vi "Excel_Insert_Text.vi"(0 "worksheet":refnum<k7>, 1 "font":T1 {"font size" format="%0.2f"; "strike through" items=["Unchanged", "Yes", "No"]; "underline" items=["Unchanged", "Yes", "No"]; "italic" items=["Unchanged", "Yes", "No"]; "bold" items=["Unchanged", "Yes", "No"]}, 3 "from template?":bool, 7 "value":string, 11 "error in (no error)":errorcluster, 12 "row":i32, 13 "column":i32, 14 "name":string) -> (15 "error out":errorcluster)   [LabVIEW 2017, in "NI_ReportGenerationToolkit.lvlib"]
uses:
  <vilib>/addons/_office/NI_ReportGenerationToolkit.lvlib
  <vilib>/addons/_office/_exclsub.llb/font.ctl
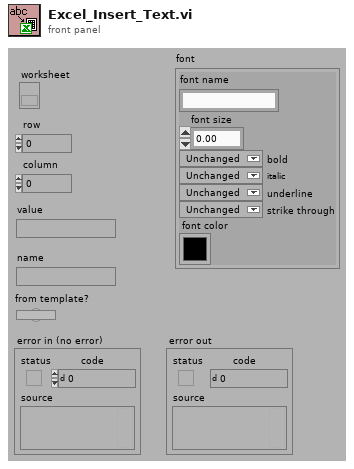
[diagram p1: front panel]
types:
  T1 = typedef "NI_ReportGenerationToolkit.lvlib/font.ctl" = cluster{"font name":string, "font size":dbl, "bold":u16, "italic":u16, "underline":u16, "strike through":u16, "font color":u32}
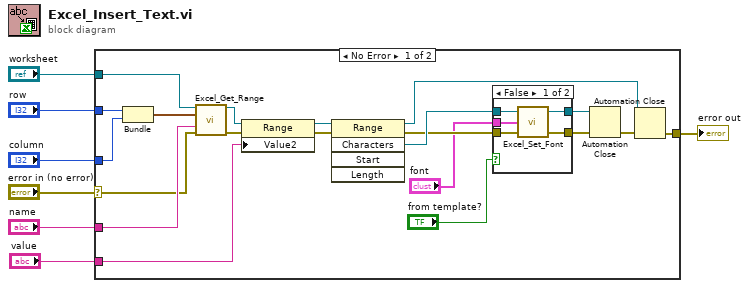
[diagram p0: block diagram]
diagram:
  n1 = case shown="No Error" "error in (no error)" {
    selector: "error in (no error)" -> [w9 w35]
    tunnel: "value" -> [w27 _]
    tunnel: [w26 w35] -> w6
    tunnel: "worksheet" -> [w15 _]
    tunnel: "column" -> [w14 _]
    tunnel: "row" -> [w13 _]
    tunnel: "name" -> [w11 _]
    frame No Error {
      n2 = Bundle("row"=w13, "column"=w14) -> (w12:cluster{"row":i32, "column":i32})  [unwired: 1 out]
      n3 = call <vilib>:"Excel_Get_Range.vi"("Excel._Worksheet"=w15, "start"=w12, "name"=w11, "error in (no error)"=w9) -> ("Range"=w16:refnum<k7>, "error out"=w17:errorcluster)  [unwired: 1 in, 9 out]
      n4 = property class="Range"(reference=w16, error in=w17, "Value2"=w27) -> (reference out=w25:refnum<k7>, error out=w24:errorcluster)
      n5 = invoke class="Range" method="Characters"(reference=w25, error in=w24) -> (reference out=w8:refnum<k7>, error out=w22:errorcluster, "Characters"=w23:refnum<k7>)  [unwired: 3 in, 2 out]
      n6 = case shown="False" "from template?" {
        tunnel: w23 -> [w32 w34]
        tunnel: w22 -> [w31 w33]
        tunnel: "font" -> [w30 _]
        tunnel: [w29 w33] -> w20
        tunnel: [w28 w34] -> w19
        frame False {
          n7 = call <vilib>:"Excel_Set_Font.vi"("Excel.Characters"=w32, "font"=w30, "error in (no error)"=w31) -> ("Excel.Characters out"=w28:refnum<k7>, "error out"=w29:errorcluster)  [unwired: 5 out]
        }
        frame True {
        }
      }
      n8 = Automation Close(3:w20, 5:w19) -> (0:w18:errorcluster)
      n9 = Automation Close(3:w18, 5:w8) -> (0:w26:errorcluster)
    }
    frame Error {
    }
  }
  "error out" <- w6
